vi "PIM XY Chart Buffer.vi"(8 "clear first (no:F)":bool, 9 "chart length (points)":i32=100, 11 "new number":dbl format="%.2f") -> (3 "new array":dbl[](array[numeric]) format="%.2f")   [LabVIEW 2011]
doc: "This reentrant VI uses an XY graph to mimic the behavior of an XY chart, in that it plots a stipulated amount of the most recently acquired data points. The chart data is stored in a static local variable of the output XY chart indicator.\n\nBecause the VI has been marked reentrant (in VI setup), you can make multiple parallel calls to the VI without confusing the memory. Use the new points array input to supply multiple points at once, or leave the array unwired (empty) and use the new point cluster input to supply one point at a time. If the locally stored chart array is not equal to chart length, it is expanded to that lenght by replicating the most recently acquired point. Data in excess of the history length is discarded. Set clear first to clear the chart history before processing the new points."
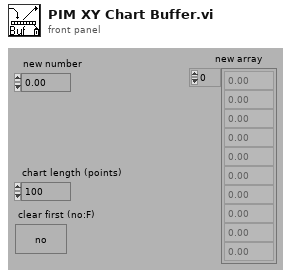
[diagram p1: front panel]
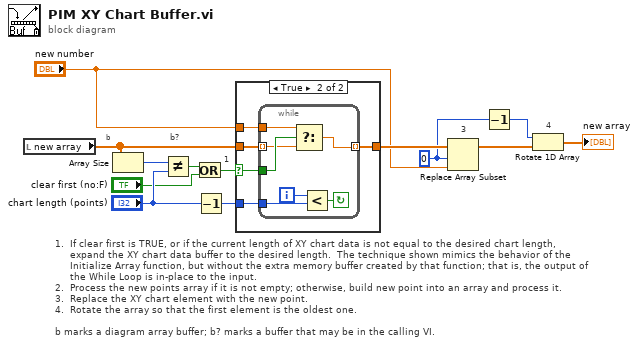
[diagram p0: block diagram]
diagram:
  w2 = 0 ("Index")
  # "3"
  # "1.  If clear first is TRUE, or if the current length of XY chart data is not equal to the desired chart length,\n     expand the XY chart data buffer to the desired length.  The technique shown mimics the behavior of the\n     Initialize Array function, but without the extra memory buffer created by that function; that is, the output of\n     the While Loop is in-place to the input.\n2.  Process the new points array if it is not empty; otherwise, build new point into an array and process it.\n3.  Replace the XY chart element with the new point.  \n4.  Rotate the array so that the first element is the oldest one.\n\nb marks a diagram array buffer; b? marks a buffer that may be in the calling VI."
  # "b"
  # "4"
  # "1"
  # "b?"
  n1 = local read "new array"() -> (w7:dbl[])
  n2 = Array Size(array=w7) -> (size(s)=w11:i32)
  n3 = Not Equal?(x=w11, y="chart length (points)") -> (x != y?=w9:bool)
  n4 = Or(x=w9, y="clear first (no:F)") -> (x .or. y?=w6:bool)
  n5 = Decrement(x="chart length (points)") -> (x-1=w8:i32)
  n6 = case shown="True" w6 {
    selector: w6 -> [_ w16]
    tunnel: [w14 w19] -> w12
    tunnel: w8 -> [_ w18]
    tunnel: w7 -> [w14 w17]
    tunnel: "new number" -> [_ w15]
    frame False {
    }
    frame True {
      n7 = while {
        tunnel: w15 -> [w20]
        tunnel: w16 -> [w23]
        tunnel: [w21] -> w19 mode=indexing
        tunnel: w18 -> [w26]
        tunnel: w17 -> [w22] mode=indexing
        i -> [w25]
        stop <- w24 continue-if-true
        n8 = Select(t=w20, s=w23, f=w22) -> (s? t:f=w21:dbl)
        n9 = Less?(x=w25, y=w26) -> (x < y?=w24:bool)
      }
    }
  }
  n10 = Replace Array Subset(array=w12, new element="new number", index=w2) -> (w5:dbl[])
  n11 = Decrement(x=w2) -> (x-1=w1:i32)
  n12 = Rotate 1D Array(1:w5, 2:w1) -> (0:→"new array":dbl[])
